vi "R45_1-RT.vi"() -> ()   [LabVIEW 2016]
uses:
  control vi/controls/Aperture states.ctl
  control vi/controls/Faraday cup states.ctl
  SCA/controls/GP307 cluster.ctl
  control vi/controls/Cryo Readback.ctl
  control vi/controls/Glassman Control.ctl
  <vilib>/FPGAPlugInAG/cRIO-9067/niLvFpga_Open_cRIO-9067.vi
  <vilib>/Utility/error.llb/Error Cluster From Error Code.vi
  <vilib>/rvi/errors/niLvFpgaAdjustHostInterfaceError.vi
  <vilib>/rvi/interface/nirviOpenFPGA/nirviOpenFPGA.xnode
  Builds/cRIOs/R45-1-cRIO/FPGA/PRIMEControl2017_FPGA-R45-1_FPGA-R45-1_ICkNri1NZgg.lvbitx
  R45_1-FPGA.vi
  <vilib>/rvi/interface/nirviReadWriteControl/nirviReadWriteControl.xnode
  control vi/controls/Faraday Cup Readback.ctl
  control vi/controls/Aperture Readback.ctl
  <vilib>/NI_Real-Time Target Support.lvlib
  NiFpgaLv.dll
panel:
  in  "Tab Control":T1(tab)
  out "Left-Steerer voltage set":dbl
  out "Right-Steerer voltage set":dbl
  out "Up-Steerer Voltage Set":dbl
  out "Down-Steerer Voltage Set":dbl
  out "Up Steerer readback.I-monitor":fxp<+/-,26,5>
  out "Up Steerer readback.V-monitor":fxp<+/-,26,7>
  out "Down Steerer readback.I-monitor":fxp<+/-,26,5>
  out "Down Steerer readback.V-monitor":fxp<+/-,26,7>
  out "Left Steerer readback.I-monitor":fxp<+/-,26,5>
  out "Left Steerer readback.V-monitor":fxp<+/-,26,7>
  out "Right Steerer readback.I-monitor":fxp<+/-,26,5>
  out "Right Steerer readback.V-monitor":fxp<+/-,26,7>
  out "Cryo status":u8[](array[numeric])
  out "Cryo On-time":u8[](array[numeric])
  out "Cryo 1st stage temp":u8[](array[numeric])
  out "2nd stage temp":u8[](array[numeric])
  out "Time since repurge":u8[](array[numeric])
  out "Status":string
  out "On-time":string
  out "1st Stage Temp":string
  out "2nd Stage Temp":string
  out "Time since re-purge":string
  out "Cryo Readback":T2
  out "Vac Cluster 1 Ion Gauge 1":u8[](array[numeric])
  out "Vac Cluster 1 Convectron 1":u8[](array[numeric])
  out "Switch Image Convectron 1":dbl
  out "Switch Image Vac Cluster":T3
  out "Switch Image Ion Gauge 1":dbl
  out "Vac Cluster 1 Ion Gauge 2":u8[](array[numeric])
  out "Vac Cluster 1 Convectron 2":u8[](array[numeric])
  out "Switch Image FC Position":cluster{"IN sensor":bool, "OUT sensor":bool}
  out "Switch Image Aperture Position":cluster{"IN sensor":bool, "OUT sensor":bool}
  out "Aperture Status":T4
  out "FC Status":T5
  out "Switch Mag Aperture actuator":bool
  out "Switch Mag FC actuator":bool
  out "Error Reporter":errorcluster
  out "Actuator-Sensor Loop error":errorcluster
  out "Cryo loop error":errorcluster
  out "Vac cluster loop error":errorcluster
  out "HV readback loop error":errorcluster
  out "HV control loop error":errorcluster
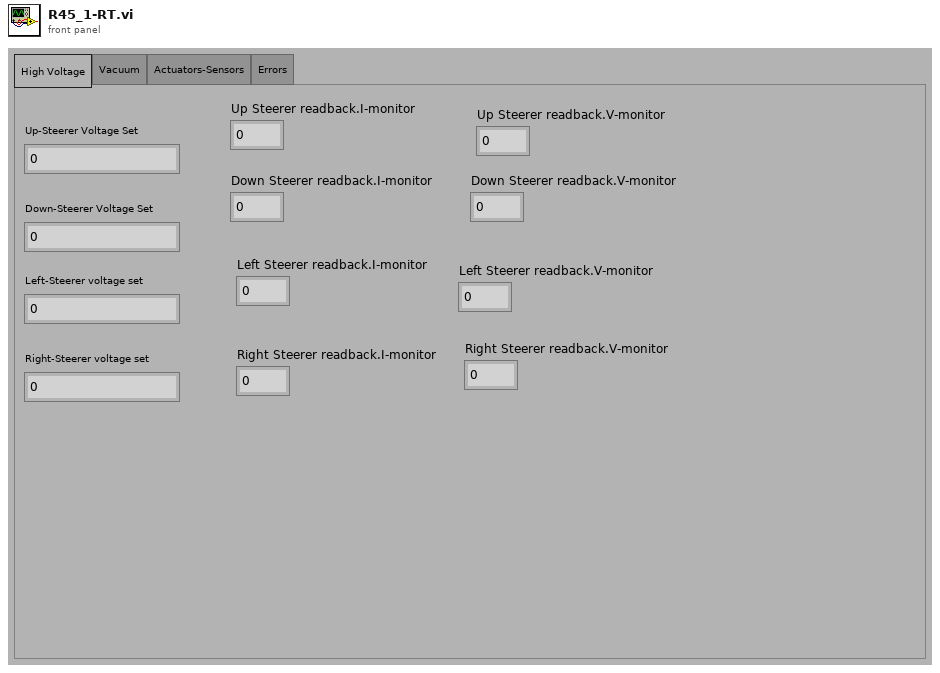
[diagram p1: front panel]
types:
  T1 = enum32{"High Voltage", "Vacuum", "Actuators-Sensors", "Errors"}
  T2 = typedef "Cryo Readback.ctl" = cluster{"Status":string, "On-time":string, "1st Stage Temp":string, "2nd Stage Temp":string, "Time since re-purge":string}
  T3 = typedef "GP307 cluster.ctl" = cluster{"Ion gauge 1":string, "Convectron  Gauge 1 ":string, "Ion Gauge 2":string, "Convectrom Gauge 2":string}
  T4 = typedef "Aperture states.ctl" = enum16{"Aperture status unclear", "Aperture in", "Aperture out"}
  T5 = typedef "Faraday cup states.ctl" = enum16{"FC status unclear", "FC in", "FC out"}
  T6 = typedef "Glassman Control.ctl" = cluster{"V-program":fxp<+/-,16,5>, "HV Enable":bool}
  T7 = typedef "Faraday Cup Readback.ctl" = cluster{"IN sensor":bool, "OUT sensor":bool}
  T8 = typedef "Aperture Readback.ctl" = cluster{"IN sensor":bool, "OUT sensor":bool}
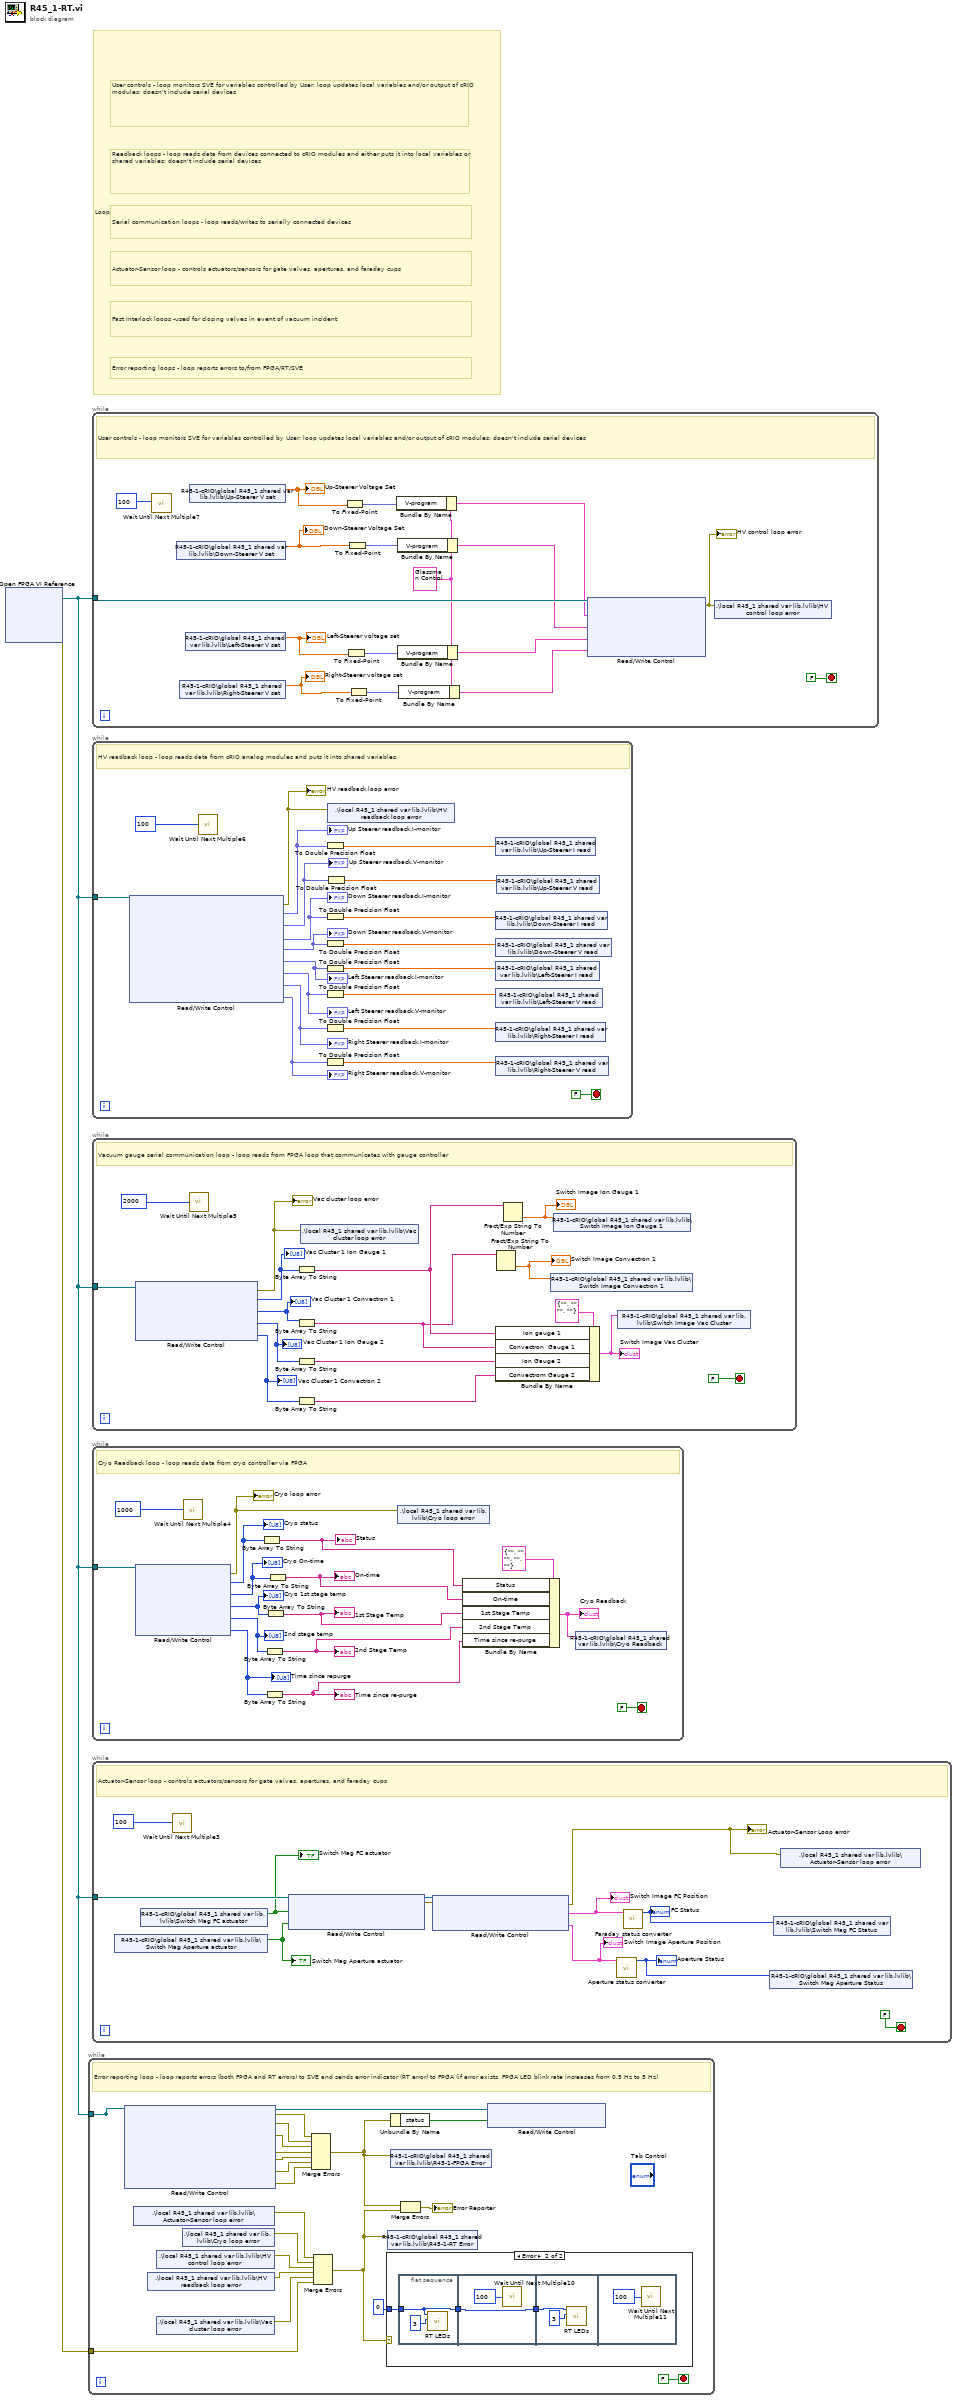
[diagram p0: block diagram]
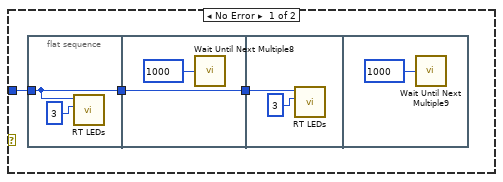
[diagram p2: hidden frame]
diagram:
  # "Actuator-Sensor loop - controls actuators/sensors for gate valves, apertures, and faraday cups"
  # "Fast Interlock loops -used for closing valves in event of vacuum incident"
  # "Error reporting loops - loop reports errors to/from FPGA/RT/SVE"
  # "Serial communication loops - loop reads/writes to serially connected devices"
  # "Readback loops - loop reads data from devices connected to cRIO modules and either puts it into local variables or shared variables; doesn't include serial devices"
  # "User controls - loop monitors SVE for variables controlled by User; loop updates local variables and/or output of cRIO modules; doesn't include serial devices"
  # "Loop legend - loops are color coded by responsibility"
  n1 = xnode "Open FPGA VI Reference"() -> ("FPGA VI Reference Out"=w2:refnum<k20>, "error out"=w1:errorcluster)  [unwired: 2 in]
  n2 = while {
    tunnel: [w23] -> _
    tunnel: w2 -> [w23]
    tunnel: w1 -> [w5]
    stop <- FALSE stop-if-true
    # "Error reporting loop - loop reports errors (both FPGA and RT errors) to SVE and sends error indicator (RT error) to FPGA (if error exists, FPGA LED blink rate increases from 0.5 Hz to 5 Hz)"
    n3 = xnode "Read/Write Control"("FPGA VI Reference In"=w23) -> ("FPGA VI Reference Out"=w14:refnum<k20>, "error out"=w22:errorcluster, "Position-Sensor readback error"=w21:errorcluster, "Cup-Aperture Control Loop Error"=w20:errorcluster, "Cryo pump error"=w19:errorcluster, "HV readback error"=w18:errorcluster, "HV Control error"=w17:errorcluster, "Vacuum Gauge 1 error"=w16:errorcluster)  [unwired: 1 in]
    n4 = shared-variable ".\\local R45_1 shared var lib.lvlib\\Actuator-Sensor loop error"() -> (w10:errorcluster)  [unwired: 1 in, 1 out]
    n5 = shared-variable ".\\local R45_1 shared var lib.lvlib\\HV readback loop error"() -> (w7:errorcluster)  [unwired: 1 in, 1 out]
    n6 = shared-variable ".\\local R45_1 shared var lib.lvlib\\HV control loop error"() -> (w8:errorcluster)  [unwired: 1 in, 1 out]
    n7 = shared-variable ".\\local R45_1 shared var lib.lvlib\\Vac cluster loop error"() -> (w6:errorcluster)  [unwired: 1 in, 1 out]
    n8 = shared-variable ".\\local R45_1 shared var lib.lvlib\\Cryo loop error"() -> (w9:errorcluster)  [unwired: 1 in, 1 out]
    n9 = Merge Errors(w22, w21, w20, w19, w18, w17, w16) -> (w15:errorcluster)
    n10 = Merge Errors(w10, w9, w8, w7, w6, w5) -> (w3:errorcluster)
    n11 = case shown="Error" w3 {
      tunnel: 0 -> [w26 w34]
      frame No Error {
        n12 = flat-sequence {
          tunnel: w26 -> [w27]
          tunnel: [w27] -> w24
          tunnel: [w29] -> w25
          tunnel: w24 -> [w29]
          tunnel: w25 -> [w31]
          frame #0 {
            n13 = call <vilib>:"RT LEDs.vi"("State"=3, "LED Num"=w27) -> ()  [unwired: 4 in, 2 out]
          }
          frame #1 {
            n14 = call "Wait Until Next Multiple8"("Count(mSec)"=u16 1000) -> ()  [unwired: 1 out]
          }
          frame #2 {
            n15 = call <vilib>:"RT LEDs.vi"("State"=3, "LED Num"=w31) -> ()  [unwired: 4 in, 2 out]
          }
          frame #3 {
            n16 = call "Wait Until Next Multiple9"("Count(mSec)"=u16 1000) -> ()  [unwired: 1 out]
          }
        }
      }
      frame Error {
        n17 = flat-sequence {
          tunnel: [w37] -> w36
          tunnel: w34 -> [w37]
          tunnel: w36 -> [w39]
          tunnel: [w39] -> w35
          tunnel: w35 -> [w41]
          frame #0 {
            n18 = call <vilib>:"RT LEDs.vi"("State"=3, "LED Num"=w37) -> ()  [unwired: 4 in, 2 out]
          }
          frame #1 {
            n19 = call "Wait Until Next Multiple10"("Count(mSec)"=u16 100) -> ()  [unwired: 1 out]
          }
          frame #2 {
            n20 = call <vilib>:"RT LEDs.vi"("State"=3, "LED Num"=w41) -> ()  [unwired: 4 in, 2 out]
          }
          frame #3 {
            n21 = call "Wait Until Next Multiple11"("Count(mSec)"=u16 100) -> ()  [unwired: 1 out]
          }
        }
      }
    }
    n22 = shared-variable "R45-1-cRIO\\global R45_1 shared var lib.lvlib\\R45-1-RT Error"(w3) -> ()  [unwired: 1 in, 1 out]
    n23 = shared-variable "R45-1-cRIO\\global R45_1 shared var lib.lvlib\\R45-1-FPGA Error"(w15) -> ()  [unwired: 1 in, 1 out]
    n24 = Unbundle By Name(w15) -> ("status"=w13:bool)
    n25 = Merge Errors(w15, w3) -> (→"Error Reporter":errorcluster)
    n26 = xnode "Read/Write Control"("FPGA VI Reference In"=w14, "RT error"=w13) -> ()  [unwired: 1 in, 2 out]
  }
  n27 = while {
    tunnel: w2 -> [w60]
    stop <- FALSE stop-if-true
    w49 = T6 {"V-program"=0.0, "HV Enable"=FALSE} ("Glassman Control")
    # "User controls - loop monitors SVE for variables controlled by User; loop updates local variables and/or output of cRIO modules; doesn't include serial devices"
    n28 = call "Wait Until Next Multiple7"("Count(mSec)"=u32 100 ("millisecond multiple")) -> ()  [unwired: 1 out]
    n29 = shared-variable "R45-1-cRIO\\global R45_1 shared var lib.lvlib\\Down-Steerer V set"() -> (w47:dbl)  [unwired: 1 in, 1 out]
    "Down-Steerer Voltage Set" <- w47
    n30 = shared-variable "R45-1-cRIO\\global R45_1 shared var lib.lvlib\\Right-Steerer V set"() -> (w45:dbl)  [unwired: 1 in, 1 out]
    "Right-Steerer voltage set" <- w45
    n31 = shared-variable "R45-1-cRIO\\global R45_1 shared var lib.lvlib\\Left-Steerer V set"() -> (w46:dbl)  [unwired: 1 in, 1 out]
    "Left-Steerer voltage set" <- w46
    n32 = shared-variable "R45-1-cRIO\\global R45_1 shared var lib.lvlib\\Up-Steerer V set"() -> (w48:dbl)  [unwired: 1 in, 1 out]
    "Up-Steerer Voltage Set" <- w48
    n33 = To Fixed-Point(number=w48) -> (fixed-point=w53:fxp<+/-,20,5>)  [unwired: 1 in]
    n34 = To Fixed-Point(number=w46) -> (fixed-point=w57:fxp<+/-,20,5>)  [unwired: 1 in]
    n35 = To Fixed-Point(number=w47) -> (fixed-point=w52:fxp<+/-,20,5>)  [unwired: 1 in]
    n36 = To Fixed-Point(number=w45) -> (fixed-point=w56:fxp<+/-,20,5>)  [unwired: 1 in]
    n37 = Bundle By Name(cluster=w49, "V-program"=w53) -> (w50:T6)
    n38 = Bundle By Name(cluster=w49, "V-program"=w52) -> (w51:T6)
    n39 = Bundle By Name(cluster=w49, "V-program"=w57) -> (w54:T6)
    n40 = Bundle By Name(cluster=w49, "V-program"=w56) -> (w55:T6)
    n41 = xnode "Read/Write Control"("FPGA VI Reference In"=w60, "Up Steerer Voltage set"=w50, "Down Steerer Voltage set"=w51, "Left Steerer Voltage set"=w54, "Right Steerer Voltage set"=w55) -> ("error out"=w58:errorcluster)  [unwired: 1 in, 1 out]
    "HV control loop error" <- w58
    n42 = shared-variable ".\\local R45_1 shared var lib.lvlib\\HV control loop error"(w58) -> ()  [unwired: 1 in, 1 out]
  }
  n43 = while {
    tunnel: w2 -> [w80]
    stop <- FALSE stop-if-true
    # "HV readback loop - loop reads data from cRIO analog modules and puts it into shared variables."
    n44 = xnode "Read/Write Control"("FPGA VI Reference In"=w80) -> ("error out"=w78:errorcluster, "Up Steerer readback.I-monitor"=w77:fxp<+/-,16,5>, "Up Steerer readback.V-monitor"=w76:fxp<+/-,16,5>, "Down Steerer readback.I-monitor"=w75:fxp<+/-,16,5>, "Down Steerer readback.V-monitor"=w74:fxp<+/-,16,5>, "Left Steerer readback.I-monitor"=w73:fxp<+/-,16,5>, "Left Steerer readback.V-monitor"=w72:fxp<+/-,16,5>, "Right Steerer readback.I-monitor"=w71:fxp<+/-,16,5>, "Right Steerer readback.V-monitor"=w70:fxp<+/-,16,5>)  [unwired: 1 in, 1 out]
    "Up Steerer readback.I-monitor" <- w77
    "Up Steerer readback.V-monitor" <- w76
    "Down Steerer readback.I-monitor" <- w75
    "Down Steerer readback.V-monitor" <- w74
    "Left Steerer readback.I-monitor" <- w73
    "Left Steerer readback.V-monitor" <- w72
    "Right Steerer readback.I-monitor" <- w71
    "Right Steerer readback.V-monitor" <- w70
    "HV readback loop error" <- w78
    n45 = call "Wait Until Next Multiple6"("Count(mSec)"=u32 100 ("millisecond multiple")) -> ()  [unwired: 1 out]
    n46 = To Double Precision Float(number=w77) -> (double precision float=w69:dbl)
    n47 = To Double Precision Float(number=w75) -> (double precision float=w66:dbl)
    n48 = To Double Precision Float(number=w74) -> (double precision float=w65:dbl)
    n49 = To Double Precision Float(number=w73) -> (double precision float=w64:dbl)
    n50 = To Double Precision Float(number=w72) -> (double precision float=w63:dbl)
    n51 = To Double Precision Float(number=w71) -> (double precision float=w62:dbl)
    n52 = To Double Precision Float(number=w70) -> (double precision float=w68:dbl)
    n53 = To Double Precision Float(number=w76) -> (double precision float=w67:dbl)
    n54 = shared-variable ".\\local R45_1 shared var lib.lvlib\\HV readback loop error"(w78) -> ()  [unwired: 1 in, 1 out]
    n55 = shared-variable "R45-1-cRIO\\global R45_1 shared var lib.lvlib\\Down-Steerer I read"(w66) -> ()  [unwired: 1 in, 1 out]
    n56 = shared-variable "R45-1-cRIO\\global R45_1 shared var lib.lvlib\\Up-Steerer I read"(w69) -> ()  [unwired: 1 in, 1 out]
    n57 = shared-variable "R45-1-cRIO\\global R45_1 shared var lib.lvlib\\Down-Steerer V read"(w65) -> ()  [unwired: 1 in, 1 out]
    n58 = shared-variable "R45-1-cRIO\\global R45_1 shared var lib.lvlib\\Left-Steerer I read"(w64) -> ()  [unwired: 1 in, 1 out]
    n59 = shared-variable "R45-1-cRIO\\global R45_1 shared var lib.lvlib\\Left-Steerer V read"(w63) -> ()  [unwired: 1 in, 1 out]
    n60 = shared-variable "R45-1-cRIO\\global R45_1 shared var lib.lvlib\\Right-Steerer I read"(w62) -> ()  [unwired: 1 in, 1 out]
    n61 = shared-variable "R45-1-cRIO\\global R45_1 shared var lib.lvlib\\Right-Steerer V read"(w68) -> ()  [unwired: 1 in, 1 out]
    n62 = shared-variable "R45-1-cRIO\\global R45_1 shared var lib.lvlib\\Up-Steerer V read"(w67) -> ()  [unwired: 1 in, 1 out]
  }
  n63 = while {
    tunnel: w2 -> [w91]
    stop <- FALSE stop-if-true
    # "Vacuum gauge serial communication loop - loop reads from FPGA loop that communicates with gauge controller"
    n64 = xnode "Read/Write Control"("FPGA VI Reference In"=w91) -> ("error out"=w84:errorcluster, "Vac Cluster 1 Ion Gauge 1"=w92:u8[], "Vac Cluster 1 Convectron 1"=w87:u8[], "Vac Cluster 1 Ion Gauge 2"=w93:u8[], "Vac Cluster 1 Convectron 2"=w94:u8[])  [unwired: 1 in, 1 out]
    "Vac Cluster 1 Ion Gauge 1" <- w92
    "Vac Cluster 1 Convectron 1" <- w87
    "Vac Cluster 1 Ion Gauge 2" <- w93
    "Vac Cluster 1 Convectron 2" <- w94
    "Vac cluster loop error" <- w84
    n65 = call "Wait Until Next Multiple5"("Count(mSec)"=u32 2000 ("millisecond multiple")) -> ()  [unwired: 1 out]
    n66 = Byte Array To String(unsigned byte array=w92) -> (string=w88:string)
    n67 = Byte Array To String(unsigned byte array=w87) -> (string=w86:string)
    n68 = Byte Array To String(unsigned byte array=w93) -> (string=w95:string)
    n69 = Byte Array To String(unsigned byte array=w94) -> (string=w96:string)
    n70 = shared-variable ".\\local R45_1 shared var lib.lvlib\\Vac cluster loop error"(w84) -> ()  [unwired: 1 in, 1 out]
    n71 = Bundle By Name(cluster=T3 {"Ion gauge 1"="", "Convectron  Gauge 1 "="", "Ion Gauge 2"="", "Convectrom Gauge 2"=""} ("Ion gauge cluster control"), "Ion gauge 1"=w88, "Convectron  Gauge 1"=w86, "Ion Gauge 2"=w95, "Convectrom Gauge 2"=w96) -> (w89:T3)
    "Switch Image Vac Cluster" <- w89
    n72 = Fract/Exp String To Number(string=w86) -> (number=w83:dbl)  [unwired: 3 in, 1 out]
    "Switch Image Convectron 1" <- w83
    n73 = Fract/Exp String To Number(string=w88) -> (number=w85:dbl)  [unwired: 3 in, 1 out]
    "Switch Image Ion Gauge 1" <- w85
    n74 = shared-variable "R45-1-cRIO\\global R45_1 shared var lib.lvlib\\Switch Image Convectron 1"(w83) -> ()  [unwired: 1 in, 1 out]
    n75 = shared-variable "R45-1-cRIO\\global R45_1 shared var lib.lvlib\\Switch Image Ion Gauge 1"(w85) -> ()  [unwired: 1 in, 1 out]
    n76 = shared-variable "R45-1-cRIO\\global R45_1 shared var lib.lvlib\\Switch Image Vac Cluster"(w89) -> ()  [unwired: 1 in, 1 out]
  }
  n77 = while {
    tunnel: w2 -> [w111]
    stop <- FALSE stop-if-true
    # "Cryo Readback loop - loop reads data from cryo controller via FPGA"
    n78 = xnode "Read/Write Control"("FPGA VI Reference In"=w111) -> ("error out"=w107:errorcluster, "Cryo status"=w108:u8[], "Cryo On-time"=w109:u8[], "Cryo 1st stage temp"=w110:u8[], "2nd stage temp"=w106:u8[], "Time since repurge"=w105:u8[])  [unwired: 1 in, 1 out]
    "Cryo status" <- w108
    "Cryo On-time" <- w109
    "Cryo 1st stage temp" <- w110
    "Cryo loop error" <- w107
    "2nd stage temp" <- w106
    "Time since repurge" <- w105
    n79 = call "Wait Until Next Multiple4"("Count(mSec)"=u32 1000 ("millisecond multiple")) -> ()  [unwired: 1 out]
    n80 = Byte Array To String(unsigned byte array=w108) -> (string=w99:string)
    "Status" <- w99
    n81 = Byte Array To String(unsigned byte array=w106) -> (string=w98:string)
    "2nd Stage Temp" <- w98
    n82 = Byte Array To String(unsigned byte array=w105) -> (string=w102:string)
    "Time since re-purge" <- w102
    n83 = Byte Array To String(unsigned byte array=w110) -> (string=w101:string)
    "1st Stage Temp" <- w101
    n84 = Byte Array To String(unsigned byte array=w109) -> (string=w100:string)
    "On-time" <- w100
    n85 = shared-variable ".\\local R45_1 shared var lib.lvlib\\Cryo loop error"(w107) -> ()  [unwired: 1 in, 1 out]
    n86 = Bundle By Name(cluster=T2 {"Status"="", "On-time"="", "1st Stage Temp"="", "2nd Stage Temp"="", "Time since re-purge"=""} ("Cryo Readback"), "Status"=w99, "On-time"=w100, "1st Stage Temp"=w101, "2nd Stage Temp"=w98, "Time since re-purge"=w102) -> (w97:T2)
    "Cryo Readback" <- w97
    n87 = shared-variable "R45-1-cRIO\\global R45_1 shared var lib.lvlib\\Cryo Readback"(w97) -> ()  [unwired: 1 in, 1 out]
  }
  n88 = while {
    tunnel: w2 -> [w124]
    stop <- FALSE stop-if-true
    # "Actuator-Sensor loop - controls actuators/sensors for gate valves, apertures, and faraday cups"
    n89 = shared-variable "R45-1-cRIO\\global R45_1 shared var lib.lvlib\\Switch Mag Aperture actuator"() -> (w114:bool)  [unwired: 1 in, 1 out]
    "Switch Mag Aperture actuator" <- w114
    n90 = shared-variable "R45-1-cRIO\\global R45_1 shared var lib.lvlib\\Switch Mag FC actuator"() -> (w115:bool)  [unwired: 1 in, 1 out]
    "Switch Mag FC actuator" <- w115
    n91 = call "Wait Until Next Multiple3"("Count(mSec)"=u32 100 ("millisecond multiple")) -> ()  [unwired: 1 out]
    n92 = xnode "Read/Write Control"("FPGA VI Reference In"=w124, "Switch Mag FC actuator"=w115, "Switch Mag Aperture actuator"=w114) -> ("FPGA VI Reference Out"=w122:refnum<k20>, "error out"=w121:errorcluster)  [unwired: 1 in]
    n93 = xnode "Read/Write Control"("FPGA VI Reference In"=w122, "error in"=w121) -> ("error out"=w116:errorcluster, "Switch Mag FC Position"=w120:T7, "Switch Mag Aperture Position"=w119:T8)  [unwired: 1 out]
    "Switch Image FC Position" <- w120
    "Switch Image Aperture Position" <- w119
    "Actuator-Sensor Loop error" <- w116
    n94 = call "Aperture status converter.vi"("Aperture Position"=w119) -> ("Aperture Status"=w118:T4)  [unwired: 10 in]
    "Aperture Status" <- w118
    n95 = call "Faraday status converter.vi"("FC Position"=w120) -> ("FC Status"=w117:T5)  [unwired: 10 in]
    "FC Status" <- w117
    n96 = shared-variable "R45-1-cRIO\\global R45_1 shared var lib.lvlib\\Switch Mag Aperture Status"(w118) -> ()  [unwired: 1 in, 1 out]
    n97 = shared-variable "R45-1-cRIO\\global R45_1 shared var lib.lvlib\\Switch Mag FC Status"(w117) -> ()  [unwired: 1 in, 1 out]
    n98 = shared-variable ".\\local R45_1 shared var lib.lvlib\\Actuator-Sensor loop error"(w116) -> ()  [unwired: 1 in, 1 out]
  }
